vi "SpinnySTOP.vi"(8 "error in":errorcluster, 9 "Stepper #":u8=1, 11 "Arduino Resource":T1={"VISA resource"="", "Board Type"=enum."Uno", "Connection Type"=enum."USB / Serial", "Bytes Per Packet (15)"=15}) -> (0 "error out":errorcluster, 3 "Arduino Resource Out":T1={"VISA resource"="", "Board Type"=enum."Uno", "Connection Type"=enum."USB / Serial", "Bytes Per Packet (15)"=15})   [LabVIEW 2014]
doc: "stop the specified stepper motor."
uses:
  <vilib>/LabVIEW Interface for Arduino/Type Defs/Arduino Resource.ctl
  <vilib>/LabVIEW Interface for Arduino/Type Defs/Board Type.ctl
  <vilib>/LabVIEW Interface for Arduino/LabVIEW Interface for Arduino.lvlib
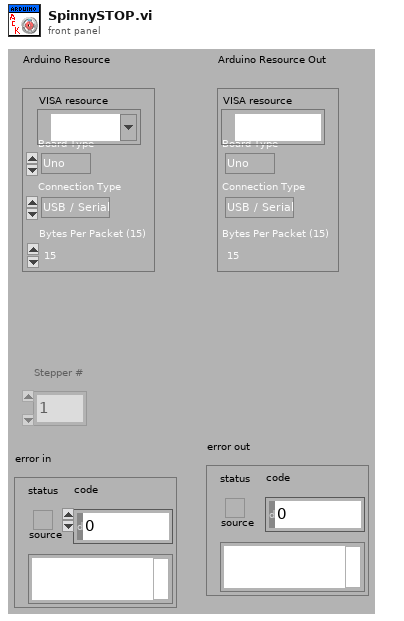
[diagram p1: front panel]
types:
  T1 = typedef "LabVIEW Interface for Arduino.lvlib/Arduino Resource.ctl" = cluster{"VISA resource":refnum<visa-resource-name>, "Board Type":T2, "Connection Type":enum8{"USB / Serial"}, "Bytes Per Packet (15)":u8}
  T2 = typedef "LabVIEW Interface for Arduino.lvlib/Board Type.ctl" = enum16{"Uno", "Dimuelanove w/Atmega 328", "Mega 2560"}
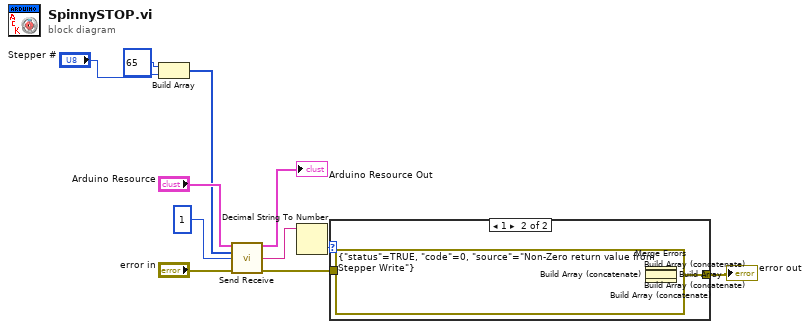
[diagram p0: block diagram]
diagram:
  n1 = Build Array(u8 65, "Stepper #") -> (w8:u8[])
  n2 = call <vilib>:"Send Receive.vi"("Arduino Resource"="Arduino Resource", "Data"=w8, "Bytes To Read (0)"=u8 1, "error in"="error in") -> ("Arduino Resource"=→"Arduino Resource Out":T1, "Read Buffer"=w2:string, "error out"=w3:errorcluster)  [unwired: 9 in]
  n3 = Decimal String To Number(string=w2) -> (number=w5:i32)  [unwired: 2 in, 1 out]
  n4 = case shown="1" w5 {
    tunnel: w3 -> [w12 w20]
    tunnel: [w12 w19] -> w4
    frame 0, Default {
    }
    frame 1 {
      n5 = Build Array(w20, errorcluster {"status"=TRUE, "code"=0, "source"="Non-Zero return value from Stepper Write"} ("error in")) -> (w17:errorcluster[])
      n6 = Build Array (concatenate)(w17) -> (w16:errorcluster[])
      n7 = Build Array (concatenate)(w16) -> (w15:errorcluster[])
      n8 = Build Array (concatenate)(w15) -> (w14:errorcluster[])
      n9 = Build Array (concatenate)(w14) -> (w13:errorcluster[])
      n10 = Merge Errors(w13) -> (w19:errorcluster)
    }
  }
  "error out" <- w4
